vi "Move-Move Command.vi"(1 "Move-SubIndex":dbl[](array[numeric]), 2 "Move-Move Command":T1=enum."SetTRF") -> ()   [LabVIEW 2018]
uses:
  Type Define/Commmands.ctl
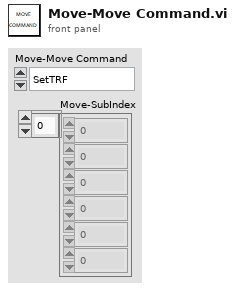
[diagram p1: front panel]
types:
  T1 = typedef "Commmands.ctl" = enum16{"No command", "Movejoints", "MovePose", "MoveLin", "MoveLinRelTRF", "MoveLinRelWRF", "Delay", "SetBlending", "SetJointVel", "SetJointAcc", "SetCartAngVel", "SetCartLinVel", "SetCartAcc", "SetTRF", "SetWRF", "SetConf", "SetAutoConf", "SetCheckpoint", "Gripper", "SetGripperVel", "SetGripperForce", "MovejointsVel", "MoveLinVelWRF", "MoveLinVelTRF", "SetVelTimeout"}
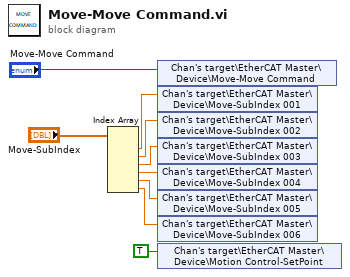
[diagram p0: block diagram]
diagram:
  n1 = Index Array(array="Move-SubIndex") -> (element #1=w9:dbl, element #2=w8:dbl, element #3=w7:dbl, element #4=w6:dbl, element #5=w5:dbl, element #6=w4:dbl)  [unwired: 6 in]
  n2 = shared-variable "Chan's target\\EtherCAT Master\\Device\\Move-Move Command"("Move-Move Command") -> ()  [unwired: 1 in, 1 out]
  n3 = shared-variable "Chan's target\\EtherCAT Master\\Device\\Move-SubIndex 001"(w9) -> ()  [unwired: 1 in, 1 out]
  n4 = shared-variable "Chan's target\\EtherCAT Master\\Device\\Move-SubIndex 002"(w8) -> ()  [unwired: 1 in, 1 out]
  n5 = shared-variable "Chan's target\\EtherCAT Master\\Device\\Move-SubIndex 003"(w7) -> ()  [unwired: 1 in, 1 out]
  n6 = shared-variable "Chan's target\\EtherCAT Master\\Device\\Move-SubIndex 004"(w6) -> ()  [unwired: 1 in, 1 out]
  n7 = shared-variable "Chan's target\\EtherCAT Master\\Device\\Move-SubIndex 005"(w5) -> ()  [unwired: 1 in, 1 out]
  n8 = shared-variable "Chan's target\\EtherCAT Master\\Device\\Move-SubIndex 006"(w4) -> ()  [unwired: 1 in, 1 out]
  n9 = shared-variable "Chan's target\\EtherCAT Master\\Device\\Motion Control-SetPoint"(TRUE ("Motion Control-SetPoint")) -> ()  [unwired: 1 in, 1 out]
